vi "Kinect Gesture Processing.vi"() -> (0 "Joystick Data":T1)   [LabVIEW 2012]
doc: "This VI imlements the framework and scheduler for your robotics program. It should not be necessary to modify the framework. You are expected to add your code to the VIs called from Robot Main, the ones located in the Team Code within the project."
uses:
  <vilib>/addons/Kinect/SkeletonVertexTrackState.ctl
  <vilib>/addons/Kinect/Skeleton Vertex Index.ctl
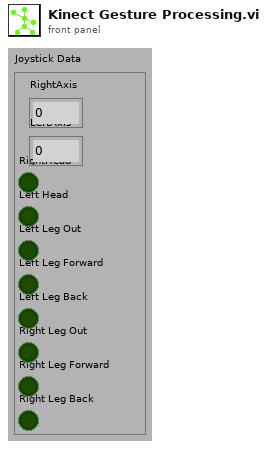
[diagram p1: front panel]
types:
  T1 = cluster{"RightAxis":dbl, "LeftAxis":dbl, "RightHead":bool, "Left Head":bool, "Left Leg Out":bool, "Left Leg Forward":bool, "Left Leg Back":bool, "Right Leg Out":bool, "Right Leg Forward":bool, "Right Leg Back":bool}
  T2 = typedef "Skeleton Vertex Index.ctl" = i32
  T3 = typedef "SkeletonVertexTrackState.ctl" = enum32{"NotTracked", "Inferred", "Tracked"}
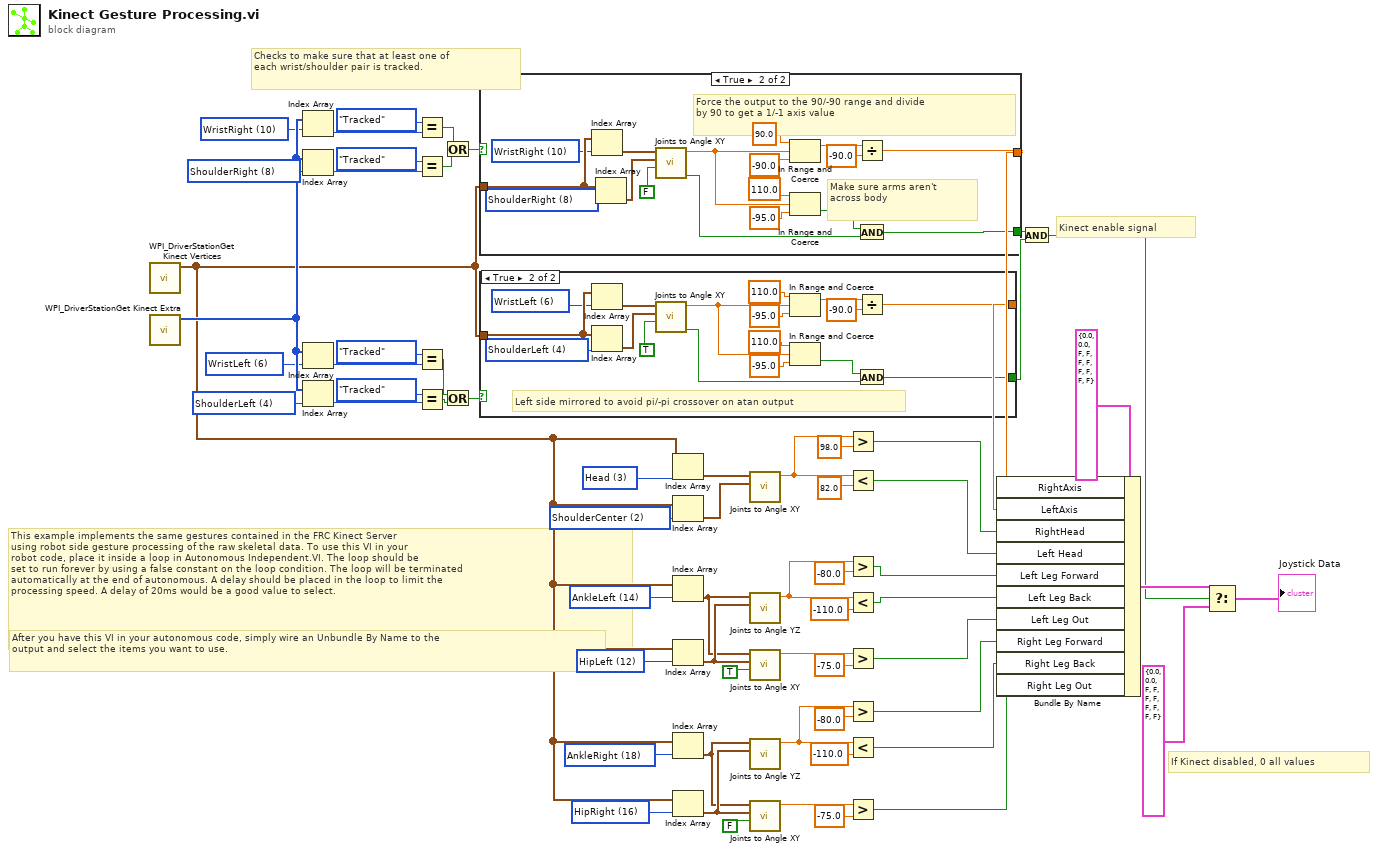
[diagram p0: block diagram]
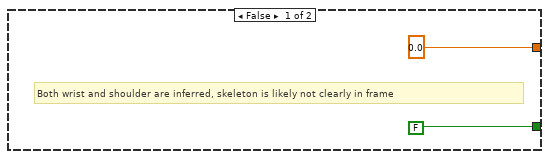
[diagram p2: hidden frame]
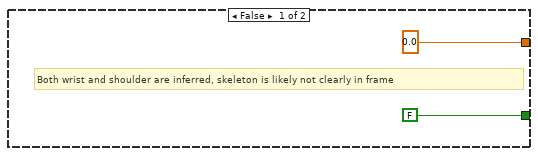
[diagram p3: hidden frame]
diagram:
  w2 = T2 16 items=["HipCenter", "Spine", "ShoulderCenter", "Head", "ShoulderLeft", "ElbowLeft", "WristLeft", "HandLeft", "ShoulderRight", "ElbowRight", "WristRight", "HandRight", "HipLeft", "KneeLeft", "AnkleLeft", "FootLeft", "HipRight", "KneeRight", "AnkleRight", "FootRight"] ("Skeleton Joints")
  w3 = T2 18 items=["HipCenter", "Spine", "ShoulderCenter", "Head", "ShoulderLeft", "ElbowLeft", "WristLeft", "HandLeft", "ShoulderRight", "ElbowRight", "WristRight", "HandRight", "HipLeft", "KneeLeft", "AnkleLeft", "FootLeft", "HipRight", "KneeRight", "AnkleRight", "FootRight"] ("Skeleton Joints")
  w1 = T2 12 items=["HipCenter", "Spine", "ShoulderCenter", "Head", "ShoulderLeft", "ElbowLeft", "WristLeft", "HandLeft", "ShoulderRight", "ElbowRight", "WristRight", "HandRight", "HipLeft", "KneeLeft", "AnkleLeft", "FootLeft", "HipRight", "KneeRight", "AnkleRight", "FootRight"] ("Skeleton Joints")
  w4 = T2 14 items=["HipCenter", "Spine", "ShoulderCenter", "Head", "ShoulderLeft", "ElbowLeft", "WristLeft", "HandLeft", "ShoulderRight", "ElbowRight", "WristRight", "HandRight", "HipLeft", "KneeLeft", "AnkleLeft", "FootLeft", "HipRight", "KneeRight", "AnkleRight", "FootRight"] ("Skeleton Joints")
  w5 = T2 2 items=["HipCenter", "Spine", "ShoulderCenter", "Head", "ShoulderLeft", "ElbowLeft", "WristLeft", "HandLeft", "ShoulderRight", "ElbowRight", "WristRight", "HandRight", "HipLeft", "KneeLeft", "AnkleLeft", "FootLeft", "HipRight", "KneeRight", "AnkleRight", "FootRight"] ("Skeleton Joints")
  w6 = T2 3 items=["HipCenter", "Spine", "ShoulderCenter", "Head", "ShoulderLeft", "ElbowLeft", "WristLeft", "HandLeft", "ShoulderRight", "ElbowRight", "WristRight", "HandRight", "HipLeft", "KneeLeft", "AnkleLeft", "FootLeft", "HipRight", "KneeRight", "AnkleRight", "FootRight"] ("Skeleton Joints")
  w8 = T2 4 items=["HipCenter", "Spine", "ShoulderCenter", "Head", "ShoulderLeft", "ElbowLeft", "WristLeft", "HandLeft", "ShoulderRight", "ElbowRight", "WristRight", "HandRight", "HipLeft", "KneeLeft", "AnkleLeft", "FootLeft", "HipRight", "KneeRight", "AnkleRight", "FootRight"] ("Skeleton Joints")
  w10 = T2 6 items=["HipCenter", "Spine", "ShoulderCenter", "Head", "ShoulderLeft", "ElbowLeft", "WristLeft", "HandLeft", "ShoulderRight", "ElbowRight", "WristRight", "HandRight", "HipLeft", "KneeLeft", "AnkleLeft", "FootLeft", "HipRight", "KneeRight", "AnkleRight", "FootRight"] ("Skeleton Joints")
  w9 = T2 8 items=["HipCenter", "Spine", "ShoulderCenter", "Head", "ShoulderLeft", "ElbowLeft", "WristLeft", "HandLeft", "ShoulderRight", "ElbowRight", "WristRight", "HandRight", "HipLeft", "KneeLeft", "AnkleLeft", "FootLeft", "HipRight", "KneeRight", "AnkleRight", "FootRight"] ("Skeleton Joints")
  w11 = T2 10 items=["HipCenter", "Spine", "ShoulderCenter", "Head", "ShoulderLeft", "ElbowLeft", "WristLeft", "HandLeft", "ShoulderRight", "ElbowRight", "WristRight", "HandRight", "HipLeft", "KneeLeft", "AnkleLeft", "FootLeft", "HipRight", "KneeRight", "AnkleRight", "FootRight"] ("Skeleton Joints")
  # "After you have this VI in your autonomous code, simply wire an Unbundle By Name to the\noutput and select the items you want to use."
  # "This example implements the same gestures contained in the FRC Kinect Server\nusing robot side gesture processing of the raw skeletal data. To use this VI in your\nrobot code, place it inside a loop in Autonomous Independent.VI. The loop should be\nset to run forever by using a false constant on the loop condition. The loop will be terminated\nautomatically at the end of autonomous. A delay should be placed in the loop to limit the \nprocessing speed. A delay of 20ms would be a good value to select."
  # "Checks to make sure that at least one of\neach wrist/shoulder pair is tracked."
  # "If Kinect disabled, 0 all values"
  # "Kinect enable signal"
  n1 = call <vilib>:"WPI_DriverStationGet Kinect Vertices.vi"() -> ("Skeleton Vertices"=w7:cluster{"x":sgl, "y":sgl, "z":sgl}[])  [unwired: 10 in, 1 out]
  n2 = call <vilib>:"WPI_DriverStationGet Kinect Extra.vi"() -> ("Skeleton Tracking State"=w29:T3[])  [unwired: 7 in, 4 out]
  n3 = Index Array(array=w29, index=w11) -> (element=w58:T3)
  n4 = Index Array(array=w29, index=w9) -> (element=w60:T3)
  n5 = Index Array(array=w29, index=w10) -> (element=w52:T3)
  n6 = Index Array(array=w29, index=w8) -> (element=w54:T3)
  n7 = Equal?(x=SkeletonVertexTrackState."Tracked", y=w58) -> (x = y?=w62:bool)
  n8 = Equal?(x=SkeletonVertexTrackState."Tracked", y=w60) -> (x = y?=w61:bool)
  n9 = Equal?(x=SkeletonVertexTrackState."Tracked", y=w52) -> (x = y?=w55:bool)
  n10 = Equal?(x=SkeletonVertexTrackState."Tracked", y=w54) -> (x = y?=w64:bool)
  n11 = Or(x=w62, y=w61) -> (x .or. y?=w63:bool)
  n12 = Or(x=w55, y=w64) -> (x .or. y?=w56:bool)
  n13 = case shown="True" w63 {
    tunnel: [0.0 w79] -> w37
    tunnel: w7 -> [_ w83]
    tunnel: [FALSE w78] -> w33
    frame False {
      # "Both wrist and shoulder are inferred, skeleton is likely not clearly in frame"
    }
    frame True {
      w67 = T2 8 items=["HipCenter", "Spine", "ShoulderCenter", "Head", "ShoulderLeft", "ElbowLeft", "WristLeft", "HandLeft", "ShoulderRight", "ElbowRight", "WristRight", "HandRight", "HipLeft", "KneeLeft", "AnkleLeft", "FootLeft", "HipRight", "KneeRight", "AnkleRight", "FootRight"] ("Skeleton Joints")
      w68 = T2 10 items=["HipCenter", "Spine", "ShoulderCenter", "Head", "ShoulderLeft", "ElbowLeft", "WristLeft", "HandLeft", "ShoulderRight", "ElbowRight", "WristRight", "HandRight", "HipLeft", "KneeLeft", "AnkleLeft", "FootLeft", "HipRight", "KneeRight", "AnkleRight", "FootRight"] ("Skeleton Joints")
      # "Make sure arms aren't\nacross body"
      # "Force the output to the 90/-90 range and divide\nby 90 to get a 1/-1 axis value"
      n14 = Index Array(array=w83, index=w68) -> (element=w76:cluster{"x":sgl, "y":sgl, "z":sgl})
      n15 = Index Array(array=w83, index=w67) -> (element=w75:cluster{"x":sgl, "y":sgl, "z":sgl})
      n16 = call "Joints to Angle XY.vi"("Mirror"=FALSE, "Origin Joint"=w75, "Moving Joint"=w76) -> ("In-Plane"=w69:bool, "Angle"=w82:dbl)  [unwired: 7 in]
      n17 = In Range and Coerce(upper limit=90.0, x=w82, lower limit=-90.0) -> (coerced(x)=w80:dbl)  [unwired: 1 out]
      n18 = In Range and Coerce(upper limit=110.0, x=w82, lower limit=-95.0) -> (In Range?=w77:bool)  [unwired: 1 out]
      n19 = Divide(x=w80, y=-90.0) -> (x/y=w79:dbl)
      n20 = And(x=w77, y=w69) -> (x .and. y?=w78:bool)
    }
  }
  n21 = case shown="True" w56 {
    tunnel: [0.0 w96] -> w36
    tunnel: w7 -> [_ w102]
    tunnel: [FALSE w92] -> w32
    frame False {
      # "Both wrist and shoulder are inferred, skeleton is likely not clearly in frame"
    }
    frame True {
      w86 = T2 4 items=["HipCenter", "Spine", "ShoulderCenter", "Head", "ShoulderLeft", "ElbowLeft", "WristLeft", "HandLeft", "ShoulderRight", "ElbowRight", "WristRight", "HandRight", "HipLeft", "KneeLeft", "AnkleLeft", "FootLeft", "HipRight", "KneeRight", "AnkleRight", "FootRight"] ("Skeleton Joints")
      w87 = T2 6 items=["HipCenter", "Spine", "ShoulderCenter", "Head", "ShoulderLeft", "ElbowLeft", "WristLeft", "HandLeft", "ShoulderRight", "ElbowRight", "WristRight", "HandRight", "HipLeft", "KneeLeft", "AnkleLeft", "FootLeft", "HipRight", "KneeRight", "AnkleRight", "FootRight"] ("Skeleton Joints")
      # "Left side mirrored to avoid pi/-pi crossover on atan output"
      n22 = Index Array(array=w102, index=w87) -> (element=w91:cluster{"x":sgl, "y":sgl, "z":sgl})
      n23 = Index Array(array=w102, index=w86) -> (element=w90:cluster{"x":sgl, "y":sgl, "z":sgl})
      n24 = call "Joints to Angle XY.vi"("Mirror"=TRUE, "Origin Joint"=w90, "Moving Joint"=w91) -> ("In-Plane"=w88:bool, "Angle"=w95:dbl)  [unwired: 7 in]
      n25 = In Range and Coerce(upper limit=110.0, x=w95, lower limit=-95.0) -> (coerced(x)=w101:dbl)  [unwired: 1 out]
      n26 = In Range and Coerce(upper limit=110.0, x=w95, lower limit=-95.0) -> (In Range?=w93:bool)  [unwired: 1 out]
      n27 = Divide(x=w101, y=-90.0) -> (x/y=w96:dbl)
      n28 = And(x=w93, y=w88) -> (x .and. y?=w92:bool)
    }
  }
  n29 = Index Array(array=w7, index=w6) -> (element=w28:cluster{"x":sgl, "y":sgl, "z":sgl})
  n30 = Index Array(array=w7, index=w5) -> (element=w27:cluster{"x":sgl, "y":sgl, "z":sgl})
  n31 = Index Array(array=w7, index=w4) -> (element=w23:cluster{"x":sgl, "y":sgl, "z":sgl})
  n32 = Index Array(array=w7, index=w1) -> (element=w24:cluster{"x":sgl, "y":sgl, "z":sgl})
  n33 = Index Array(array=w7, index=w3) -> (element=w25:cluster{"x":sgl, "y":sgl, "z":sgl})
  n34 = Index Array(array=w7, index=w2) -> (element=w26:cluster{"x":sgl, "y":sgl, "z":sgl})
  n35 = call "Joints to Angle XY.vi"("Origin Joint"=w27, "Moving Joint"=w28) -> ("Angle"=w44:dbl)  [unwired: 8 in, 1 out]
  n36 = call "Joints to Angle YZ.vi"("Origin Joint"=w24, "Moving Joint"=w23) -> ("Angle"=w47:dbl)  [unwired: 9 in]
  n37 = call "Joints to Angle XY.vi"("Mirror"=TRUE, "Origin Joint"=w24, "Moving Joint"=w23) -> ("Angle"=w48:dbl)  [unwired: 7 in, 1 out]
  n38 = call "Joints to Angle YZ.vi"("Origin Joint"=w26, "Moving Joint"=w25) -> ("Angle"=w22:dbl)  [unwired: 9 in]
  n39 = call "Joints to Angle XY.vi"("Mirror"=FALSE, "Origin Joint"=w26, "Moving Joint"=w25) -> ("Angle"=w39:dbl)  [unwired: 7 in, 1 out]
  n40 = Greater?(x=w44, y=98.0) -> (0:w35:bool)
  n41 = Less?(x=w44, y=82.0) -> (x < y?=w34:bool)
  n42 = Greater?(x=w47, y=-80.0) -> (0:w20:bool)
  n43 = Less?(x=w47, y=-110.0) -> (x < y?=w19:bool)
  n44 = Greater?(x=w48, y=-75.0) -> (0:w18:bool)
  n45 = Greater?(x=w22, y=-80.0) -> (0:w17:bool)
  n46 = Less?(x=w22, y=-110.0) -> (x < y?=w16:bool)
  n47 = Greater?(x=w39, y=-75.0) -> (0:w15:bool)
  n48 = Bundle By Name(cluster=T1 {"RightAxis"=0.0, "LeftAxis"=0.0, "RightHead"=FALSE, "Left Head"=FALSE, "Left Leg Out"=FALSE, "Left Leg Forward"=FALSE, "Left Leg Back"=FALSE, "Right Leg Out"=FALSE, "Right Leg Forward"=FALSE, "Right Leg Back"=FALSE} ("f"), "RightAxis"=w37, "LeftAxis"=w36, "RightHead"=w35, "Left Head"=w34, "Left Leg Forward"=w20, "Left Leg Back"=w19, "Left Leg Out"=w18, "Right Leg Forward"=w17, "Right Leg Back"=w16, "Right Leg Out"=w15) -> (w31:T1)
  n49 = And(x=w33, y=w32) -> (x .and. y?=w30:bool)
  n50 = Select(t=w31, s=w30, f=T1 {"RightAxis"=0.0, "LeftAxis"=0.0, "RightHead"=FALSE, "Left Head"=FALSE, "Left Leg Out"=FALSE, "Left Leg Forward"=FALSE, "Left Leg Back"=FALSE, "Right Leg Out"=FALSE, "Right Leg Forward"=FALSE, "Right Leg Back"=FALSE}) -> (s? t:f=→"Joystick Data":T1)
